vi "fgvFsmTemplate.vi"(7 "Urgent":bool, 8 "Error In":errorcluster caption="에러 입력", 10 "Write":T1, 11 "Function":T2) -> (0 "Error Out":errorcluster caption="에러 출력", 2 "Read":T1, 3 "Count":i32)   [LabVIEW 2018]
uses:
  controls/enumFgvFunctionFsm.ctl
  enumFsmTemplate.ctl
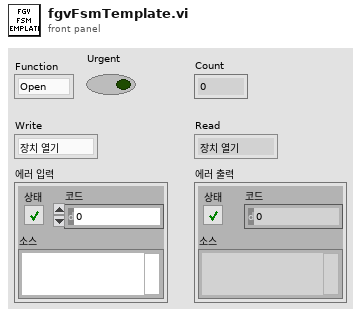
[diagram p1: front panel]
types:
  T1 = typedef "enumFsmTemplate.ctl" = enum16{"장치 열기", "장치 설정", "장치 읽기", "장치 쓰기", "장치 닫기", "대기", "에러"}
  T2 = typedef "enumFgvFunctionFsm.ctl" = enum16{"Open", "Read", "Check", "Clear", "Write", "Close"}
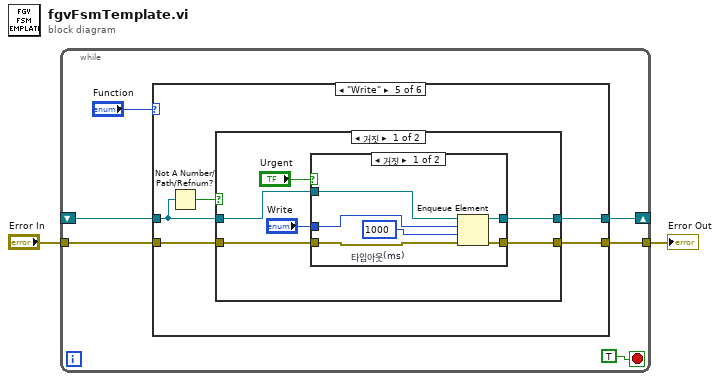
[diagram p0: block diagram]
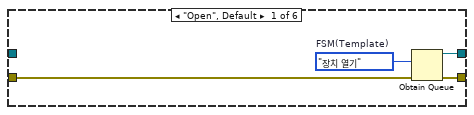
[diagram p2: hidden frame]
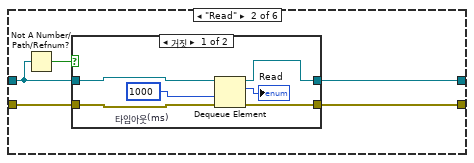
[diagram p3: hidden frame]
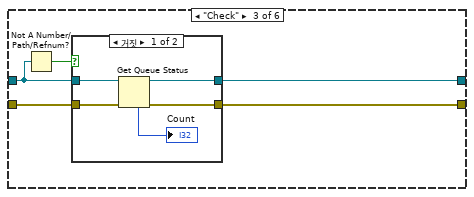
[diagram p5: hidden frame]
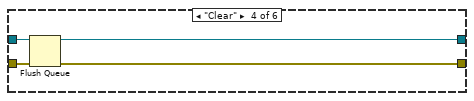
[diagram p7: hidden frame]
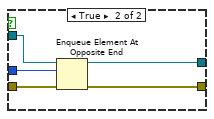
[diagram p8: hidden frame]
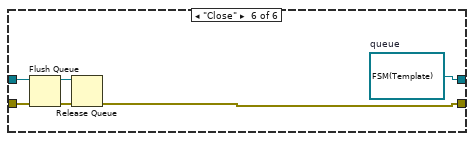
[diagram p10: hidden frame]
diagram:
  n1 = while {
    shift-right: [w6] -> _
    shift-left: _ -> [w7]
    tunnel: "Error In" -> [w5]
    tunnel: [w4] -> w1
    stop <- TRUE stop-if-true
    n2 = case shown="\"Write\"" "Function" {
      tunnel: w7 -> [_ w14 w26 w41 w43 w71]
      tunnel: [w12 w17 w30 w39 w46 w66] -> w6
      tunnel: w5 -> [w10 w16 w29 w40 w45 w69]
      tunnel: [w11 w15 w28 w38 w44 w67] -> w4
      frame "Open", Default {
        w9 = enumFsmTemplate."장치 열기"  # FSM(Template)
        n3 = Obtain Queue(element data type=w9, error in (no error)=w10) -> (queue out=w12:refnum<queue>, error out=w11:errorcluster)  [unwired: 3 in, 1 out]
      }
      frame "Read" {
        n4 = Not A Number/Path/Refnum?(number/path/refnum=w14) -> (NaN/Path/Refnum?=w13:bool)
        n5 = case shown="거짓" w13 {
          tunnel: [w23 w25] -> w17
          tunnel: w16 -> [w22 w24]
          tunnel: [w21 w24] -> w15
          tunnel: w14 -> [w19 w25]
          frame False {
            w20 = 1000  # 타임아웃(ms)
            n6 = Dequeue Element(queue=w19, timeout in ms (-1)=w20, error in (no error)=w22) -> (queue out=w23:refnum<queue>, element=→"Read":T1, error out=w21:errorcluster)  [unwired: 1 out]
          }
          frame True {
          }
        }
      }
      frame "Check" {
        n7 = Not A Number/Path/Refnum?(number/path/refnum=w26) -> (NaN/Path/Refnum?=w27:bool)
        n8 = case shown="거짓" w27 {
          tunnel: w26 -> [w35 w37]
          tunnel: [w34 w37] -> w30
          tunnel: w29 -> [w32 w36]
          tunnel: [w31 w36] -> w28
          frame False {
            n9 = Get Queue Status(queue=w35, error in (no error)=w32) -> (queue out=w34:refnum<queue>, error out=w31:errorcluster, # elements in queue=→"Count":i32)  [unwired: 1 in, 5 out]
          }
          frame True {
          }
        }
      }
      frame "Clear" {
        n10 = Flush Queue(queue=w41, error in (no error)=w40) -> (queue out=w39:refnum<queue>, error out=w38:errorcluster)  [unwired: 1 out]
      }
      frame "Write" {
        n11 = Not A Number/Path/Refnum?(number/path/refnum=w43) -> (NaN/Path/Refnum?=w42:bool)
        n12 = case shown="거짓" w42 {
          tunnel: [w52 w65] -> w46
          tunnel: w45 -> [w51 w64]
          tunnel: [w50 w64] -> w44
          tunnel: w43 -> [w49 w65]
          frame False {
            n13 = case shown="거짓" "Urgent" {
              tunnel: [w58 w60] -> w52
              tunnel: w51 -> [w57 w63]
              tunnel: [w56 w62] -> w50
              tunnel: w49 -> [w54 w61]
              tunnel: "Write" -> [w53 w59]
              frame False {
                w55 = 1000  # 타임아웃(ms)
                n14 = Enqueue Element(queue=w54, element=w53, timeout in ms (-1)=w55, error in (no error)=w57) -> (queue out=w58:refnum<queue>, error out=w56:errorcluster)  [unwired: 1 out]
              }
              frame True {
                n15 = Enqueue Element At Opposite End(queue=w61, element=w59, error in (no error)=w63) -> (queue out=w60:refnum<queue>, error out=w62:errorcluster)  [unwired: 1 in, 1 out]
              }
            }
          }
          frame True {
          }
        }
      }
      frame "Close" {
        w66 = refnum<queue> refnum items=["장치 열기", "장치 설정", "장치 읽기", "장치 쓰기", "장치 닫기", "대기", "에러"]  # queue
        n16 = Flush Queue(queue=w71, error in (no error)=w69) -> (queue out=w70:refnum<queue>, error out=w68:errorcluster)  [unwired: 1 out]
        n17 = Release Queue(queue=w70, error in (no error)=w68) -> (error out=w67:errorcluster)  [unwired: 1 in, 2 out]
      }
    }
  }
  "Error Out" <- w1
